vi "BuildCallChainString.vi"(4 "Lower levels to omit":i32 caption="Lower levels to omit (0)") -> (1 "Call chain string":string)   [LabVIEW 2017, in "GPError.lvlib"]
doc: "Builds a <B>Call chain string</B> of the format 'Top-level VI'->...->'Lowest-level VI'.\n\nBy specifying <B>Lower levels to omit</B> you can configure how much of the low end of the call chain that should be omitted, in case you embed this VI inside a more top-level function that should receive the blame.\n\nThis VI is inlined.\n\nSteen Schmidt\nGPower\n10/7 2013"
uses:
  GPError.lvlib
panel:
  # "Copyright © 2013\nSteen Schmidt, GPower\nSee enclosed license file for terms and conditions"
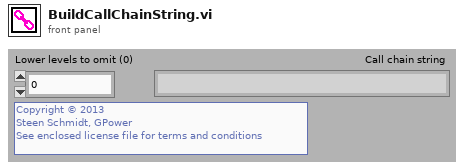
[diagram p1: front panel]
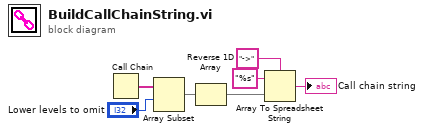
[diagram p0: block diagram]
diagram:
  n1 = Call Chain() -> (call chain=w4:string[])
  n2 = Array Subset(array=w4, index="Lower levels to omit") -> (w2:string[])  [unwired: 1 in]
  n3 = Reverse 1D Array(array=w2) -> (reversed array=w1:string[])
  n4 = Array To Spreadsheet String(delimiter (Tab)="->", array=w1, 3:"%s" ("format string")) -> (spreadsheet string=→"Call chain string":string)
